vi "GEOM_ROICorrections.vi"(9 "ROIS":T1(array[cluster]), 10 "amplifiers":T2[](array[typedef]) {"fliped" items=["none", "horizontal", "vertical"]; "type" items=["LL", "LR", "UL", "UR"]}, 11 "CorrectionType":T6) -> (1 "Corrected ROIs":T1(array[cluster]))   [LabVIEW 2016]
uses:
  GEOM_ROICorrection.ctl
  GEOM_Amplifier.ctl
  GEOM_AmpType.ctl
  GEOM_ROI.ctl
  GEOM_Coords.ctl
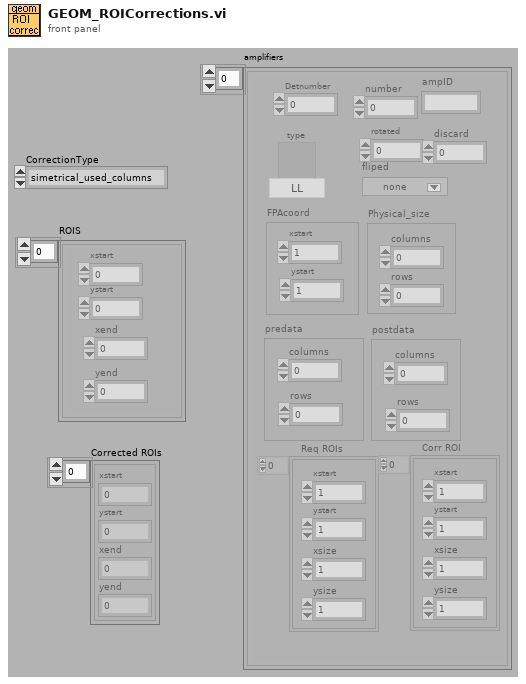
[diagram p1: front panel]
types:
  T1 = cluster{"xstart":i32, "ystart":i32, "xend":i32, "yend":i32}[]
  T2 = typedef "GEOM_Amplifier.ctl" = cluster{"number":i32, "type":T3, "rotated":i16, "fliped":u16, "FPAcoord":cluster{"xstart":i32, "ystart":i32}, "Physical_size":cluster{"columns":i32, "rows":i32}, "predata":cluster{"columns":i32, "rows":i32}, "postdata":cluster{"columns":i32, "rows":i32}, "Req ROIs":T4, "Corr ROI":T4, "Detnumber":i32, "ampID":string, "discard":i32}
  T3 = typedef "GEOM_AmpType.ctl" = u16
  T4 = typedef "GEOM_ROI.ctl" = T5[]
  T5 = typedef "GEOM_Coords.ctl" = cluster{"xstart":u32, "ystart":u32, "xsize":u32, "ysize":u32}
  T6 = typedef "GEOM_ROICorrection.ctl" = enum16{"simetrical_used_columns", "simetrical_all_columns"}
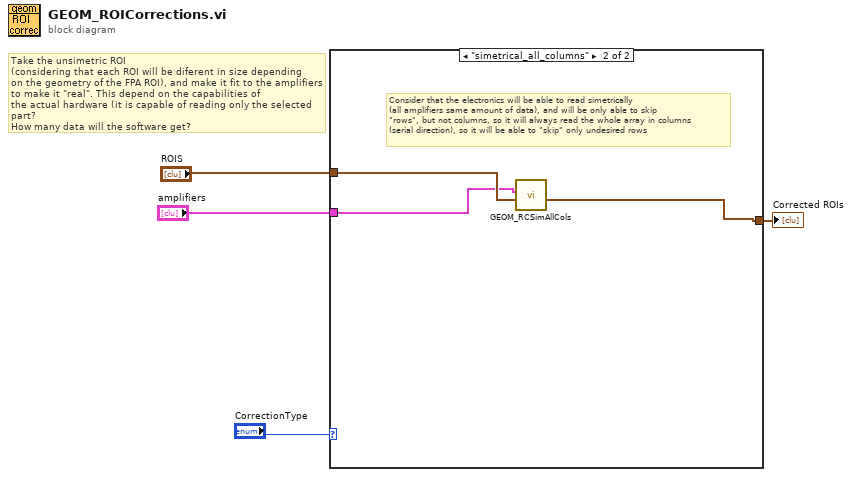
[diagram p0: block diagram]
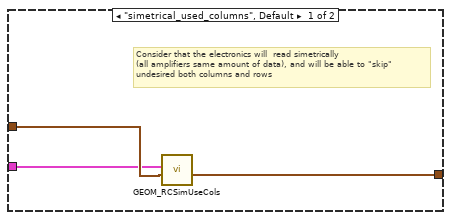
[diagram p2: hidden frame]
diagram:
  # "Take the unsimetric ROI\n(considering that each ROI will be diferent in size depending\non the geometry of the FPA ROI), and make it fit to the amplifiers\nto make it \"real\". This depend on the capabilities of\nthe actual hardware (it is capable of reading only the selected part?\nHow many data will the software get?"
  n1 = case shown="\"simetrical_all_columns\"" "CorrectionType" {
    tunnel: "amplifiers" -> [w6 w8]
    tunnel: "ROIS" -> [w7 w10]
    tunnel: [w5 w9] -> w1
    frame "simetrical_used_columns", Default {
      # "Consider that the electronics will  read simetrically\n(all amplifiers same amount of data), and will be able to \"skip\"  \nundesired both columns and rows"
      n2 = call "GEOM_RCSimUseCols.vi"("ROIS"=w7, "amplifiers"=w6) -> ("Corrected ROIs"=w5:T1)  [unwired: 9 out]
    }
    frame "simetrical_all_columns" {
      # "Consider that the electronics will be able to read simetrically\n(all amplifiers same amount of data), and will be only able to skip\n\"rows\", but not columns, so it will always read the whole array in columns\n(serial direction), so it will be able to \"skip\" only undesired rows"
      n3 = call "GEOM_RCSimAllCols.vi"("ROIS"=w10, "amplifiers"=w8) -> ("Corrected ROIs"=w9:T1)  [unwired: 9 out]
    }
  }
  "Corrected ROIs" <- w1
